vi "ColorCheck.vi"(8 "error in":errorcluster, 9 "Ignore 2":dbl=-1.0, 10 "Ignore 1":dbl=-1.0) -> (0 "error out":errorcluster, 2 "Color Id":i32)   [LabVIEW 2018]
uses:
  <vilib>/vision/NI_Vision_Development_Module.lvlib
  <vilib>/vision/driver/NI_Vision_Acquisition_Software.lvlib
  <resource>/objmgr/imaqdx.rc
panel:
  out "max index(es)":i32
  out "Color Spectrum":dbl[](array[numeric]) format="%.2f"
  out "Image Out":T1(plugin-control)
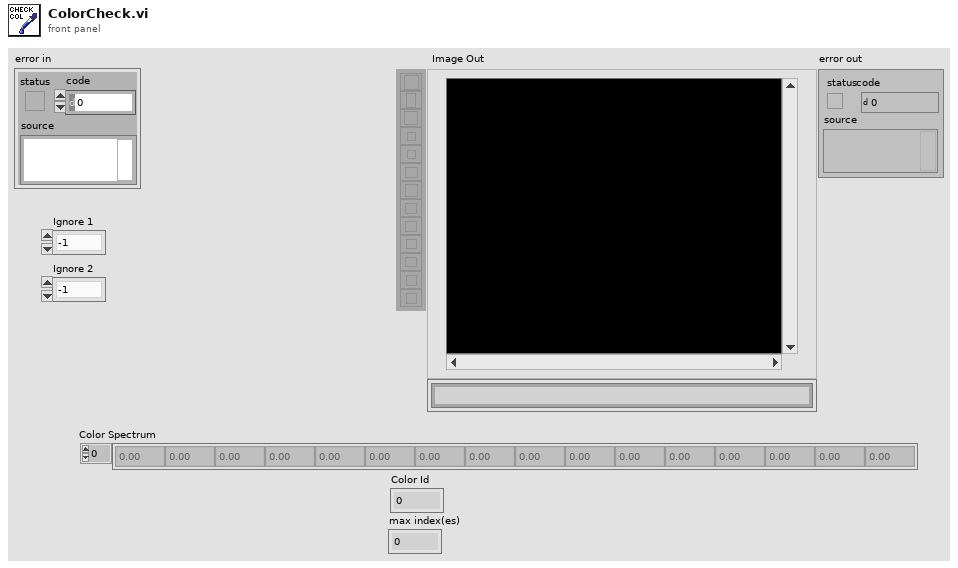
[diagram p1: front panel]
types:
  T1 = typedef "IMAQ Image.ctl" = refnum<image>
  T2 = typedef "ROI Descriptor" = cluster{"Global Rectangle":i32[], "Contours":cluster{"ID":enum32{"External", "Internal"}, "Type":u32, "Coordinates":i32[]}[]}
  T3 = typedef "IMAQdx.ctl" = refnum<k21>
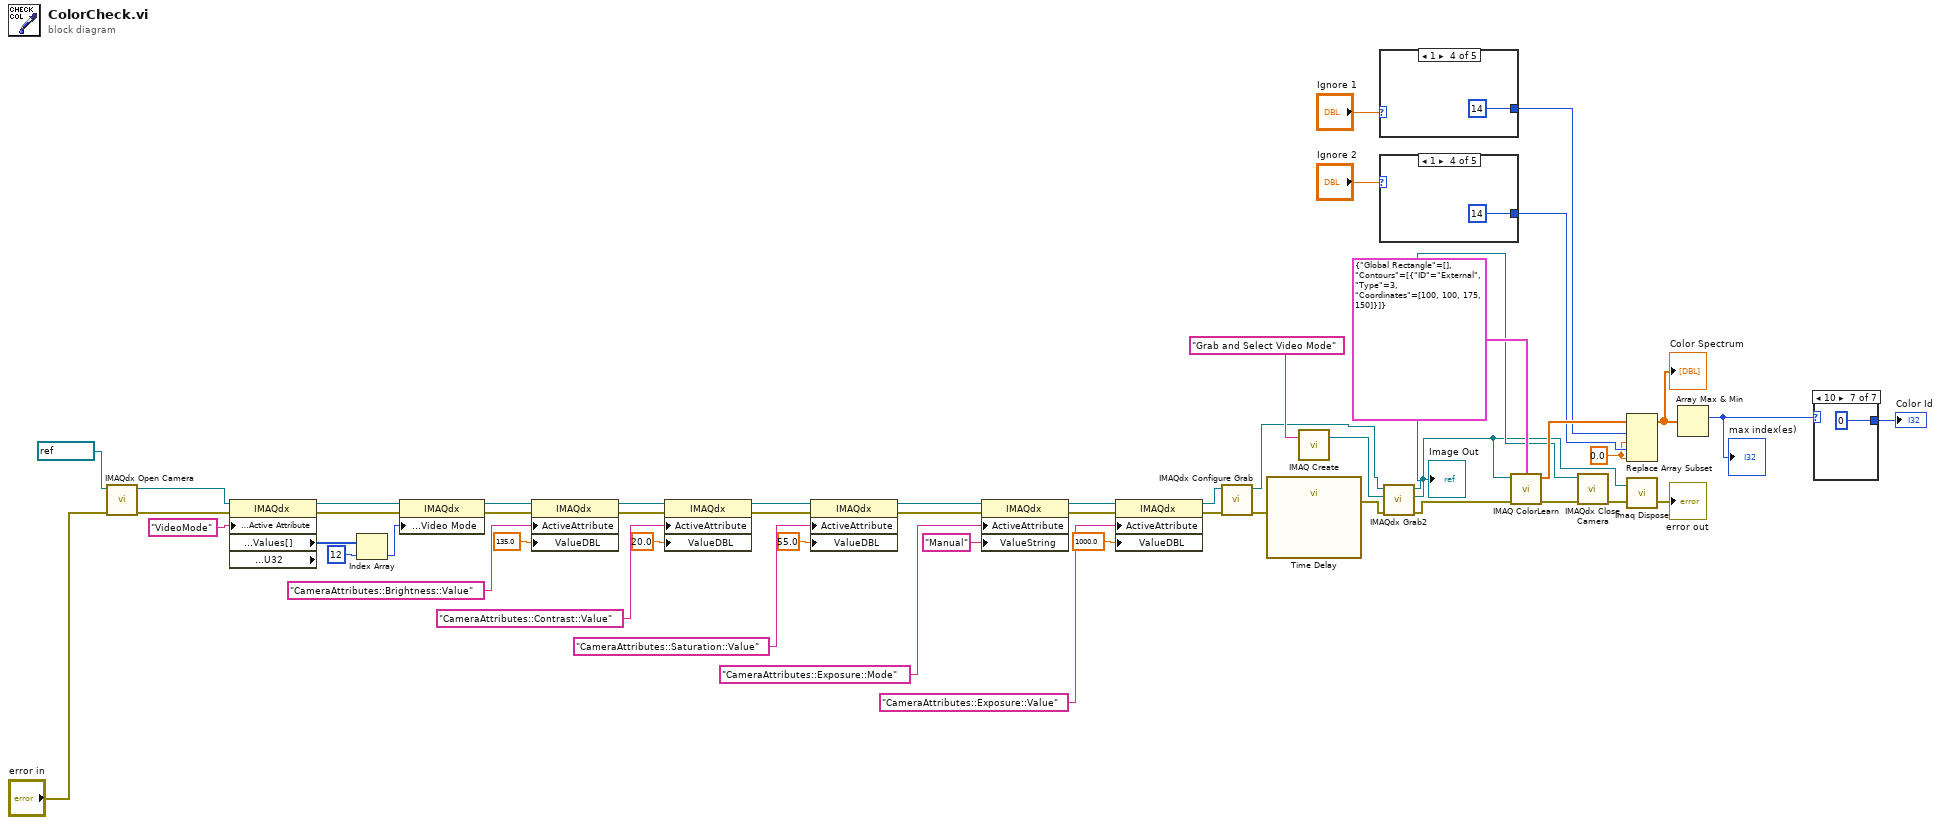
[diagram p0: block diagram]
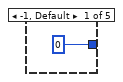
[diagram p2: hidden frame]
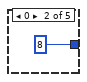
[diagram p3: hidden frame]
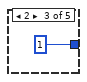
[diagram p4: hidden frame]
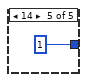
[diagram p5: hidden frame]
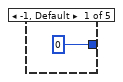
[diagram p6: hidden frame]
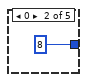
[diagram p7: hidden frame]
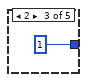
[diagram p8: hidden frame]
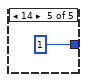
[diagram p9: hidden frame]
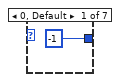
[diagram p10: hidden frame]
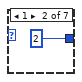
[diagram p11: hidden frame]
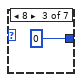
[diagram p12: hidden frame]
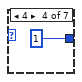
[diagram p13: hidden frame]
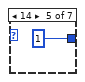
[diagram p14: hidden frame]
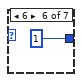
[diagram p15: hidden frame]
diagram:
  w44 = 0.0 ("new element/subarray")
  n1 = call <vilib>:"IMAQdx Open Camera.vi"("error in"="error in", "Session In"=refnum<k21> "cam0" ("Camera Name")) -> ("error out"=w13:errorcluster, "Session Out"=w15:T3)  [unwired: 1 in, 7 out]
  n2 = property class="IMAQdx" props=["Camera Attributes:Active Attribute", "Camera Attributes:Enum:Values[]", "Camera Attributes:Value:U32"](reference=w15, error in=w13, "Camera Attributes:Active Attribute"="VideoMode" ("ActiveAttribute")) -> (reference out=w18:T3, error out=w19:errorcluster, "Camera Attributes:Enum:Values[]"=w22:u32[])  [unwired: 1 out]
  n3 = Index Array(array=w22, index=12 ("Video Modes")) -> (element=w21:u32)
  n4 = property class="IMAQdx"(reference=w18, error in=w19, "Acquisition Attributes:Video Mode"=w21) -> (reference out=w25:T3, error out=w26:errorcluster)
  n5 = property class="IMAQdx"(reference=w25, error in=w26, "ActiveAttribute"="CameraAttributes::Brightness::Value", "ValueDBL"=135.0) -> (reference out=w29:T3, error out=w30:errorcluster)
  n6 = property class="IMAQdx"(reference=w29, error in=w30, "ActiveAttribute"="CameraAttributes::Contrast::Value", "ValueDBL"=20.0) -> (reference out=w31:T3, error out=w32:errorcluster)
  n7 = property class="IMAQdx"(reference=w31, error in=w32, "ActiveAttribute"="CameraAttributes::Saturation::Value", "ValueDBL"=55.0) -> (reference out=w34:T3, error out=w35:errorcluster)
  n8 = property class="IMAQdx"(reference=w34, error in=w35, "ActiveAttribute"="CameraAttributes::Exposure::Mode", "ValueString"="Manual") -> (reference out=w38:T3, error out=w39:errorcluster)
  n9 = property class="IMAQdx"(reference=w38, error in=w39, "ActiveAttribute"="CameraAttributes::Exposure::Value", "ValueDBL"=1000.0) -> (reference out=w42:T3, error out=w43:errorcluster)
  n10 = call <vilib>:"IMAQdx Configure Grab.vi"("error in"=w43, "Session In"=w42) -> ("error out"=w11:errorcluster, "Session Out"=w5:T3)  [unwired: 8 in]
  n11 = call "Time Delay"("error in (no error)"=w11) -> ("error out"=w7:errorcluster)  [unwired: 10 in]
  n12 = call "IMAQ Create"("Image Name"="Grab and Select Video Mode") -> ("New Image"=w4:T1)  [unwired: 3 in, 2 out]
  n13 = case shown="1" "Ignore 1" {
    tunnel: [0 8 1 14 1] -> w48
    frame -1, Default {
    }
    frame 0 {
    }
    frame 2 {
    }
    frame 1 {
    }
    frame 14 {
    }
  }
  n14 = case shown="1" "Ignore 2" {
    tunnel: [0 8 1 14 1] -> w45
    frame -1, Default {
    }
    frame 0 {
    }
    frame 2 {
    }
    frame 1 {
    }
    frame 14 {
    }
  }
  n15 = call <vilib>:"IMAQdx Grab2.vi"("error in"=w7, "Image In"=w4, "Session In"=w5) -> ("error out"=w6:errorcluster, "Image Out"=w2:T1, "Session Out"=w3:T3)  [unwired: 5 in, 1 out]
  "Image Out" <- w2
  n16 = call "IMAQ ColorLearn"("ROI Descriptor"=T2 {"Global Rectangle"=[], "Contours"=[{"ID"=enum."External", "Type"=3, "Coordinates"=[100, 100, 175, 150]}]}, "Image"=w2, "error in (no error)"=w6) -> ("Color Spectrum"=w49:dbl[], "error out"=w8:errorcluster)  [unwired: 5 in]
  n17 = call <vilib>:"IMAQdx Close Camera.vi"("error in"=w8, "Session In"=w3) -> ("error out"=w10:errorcluster)  [unwired: 9 out]
  n18 = Replace Array Subset(array=w49, new element #1=w44, index #1=w48, new element #2=w44, index #2=w45) -> (w47:dbl[])
  "Color Spectrum" <- w47
  n19 = call "Imaq Dispose"("Image"=w2, "error in (no error)"=w10) -> ("error out"=→"error out":errorcluster)  [unwired: 4 in]
  n20 = Array Max & Min(array=w47) -> (max index (indices)=w52:i32)  [unwired: 3 out]
  "max index(es)" <- w52
  n21 = case shown="10" w52 {
    tunnel: [-1 2 0 1 1 1 0] -> w51
    frame 0, Default {
    }
    frame 1 {
    }
    frame 8 {
    }
    frame 4 {
    }
    frame 14 {
    }
    frame 6 {
    }
    frame 10 {
    }
  }
  "Color Id" <- w51
